vi "TemperatureConversion.vi"() -> ()   [LabVIEW 2020]
panel:
  in  "Stop":bool
  out "Fahrenheit":dbl
  in  "Celsius":dbl
  # "Sample Text"
  # "Temperature Conversion"
  # "Celcius to Fahrenheit"
  # "1. The celcius is given as the input.\n2. Then Fahrenheit will appear in the side indicator"
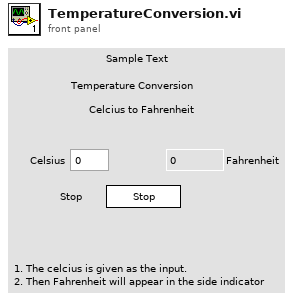
[diagram p1: front panel]
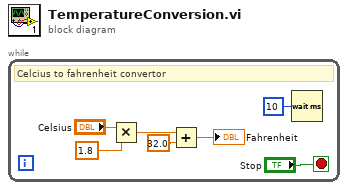
[diagram p0: block diagram]
diagram:
  n1 = while {
    stop <- "Stop" stop-if-true
    # "Celcius to fahrenheit convertor"
    n2 = Multiply(x="Celsius", y=1.8) -> (x*y=w5:dbl)
    n3 = Add(x=w5, y=32.0) -> (x+y=→"Fahrenheit":dbl)
    n4 = Wait (ms)(milliseconds to wait=u32 10) -> ()  [unwired: 1 out]
  }
